vi "G#Object_NewObject.vi"(0 "reference in":refnum<class "G#Object.lvclass">, 1 "object name (\"\")":string, 2 "user counter (T)":bool=TRUE, 3 "no registration (F)":bool, 5 "error in (no error)":errorcluster, 6 "create method":T1) -> (14 "reference out":refnum<class "G#Object.lvclass">, 15 "created new?":bool, 19 "error out":errorcluster)   [LabVIEW 2020, in "G#Object.lvclass"]
doc: "Creates a new object and registers it."
uses:
  <vilib>/addons/_AddQ/G#Object/G#Object.lvclass
  <vilib>/addons/_AddQ/G#Object/utils/G#Object_CreateMethod.ctl
  <vilib>/addons/_AddQ/G#Object/utils/G#Object_State.ctl
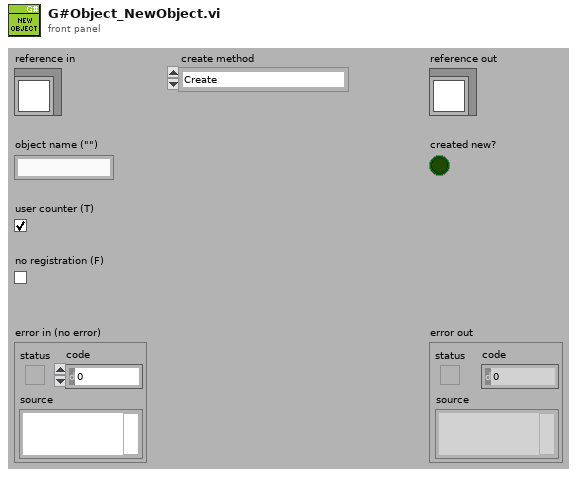
[diagram p1: front panel]
types:
  T1 = typedef "G#Object.lvclass/G#Object_CreateMethod.ctl" = enum16{"Create", "Create or look up existing", "Look up existing"}
  T2 = typedef "G#Object.lvclass/G#Object_State.ctl" = enum16{"Clear", "Create", "Delete", "Get class attributes", "Class hierarchy", "Get attribute value", "Set attribute value"}
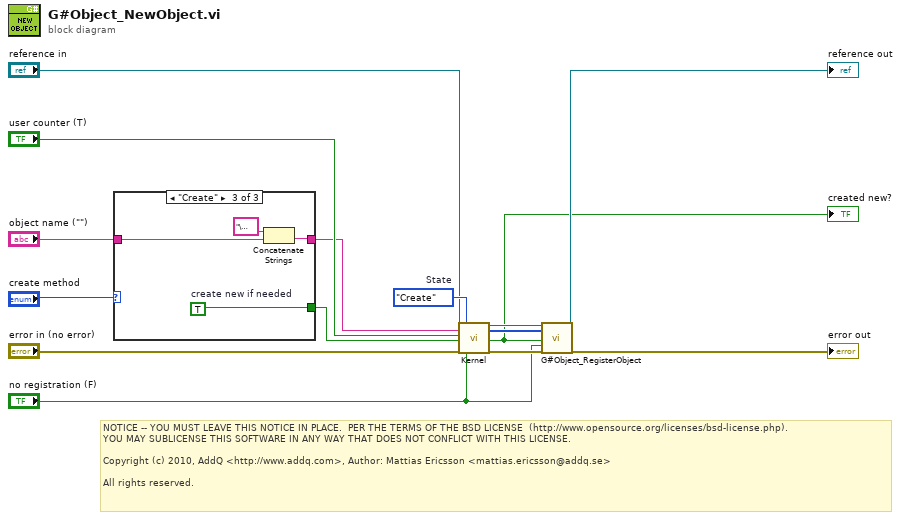
[diagram p0: block diagram]
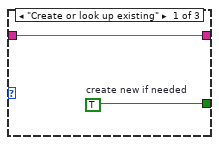
[diagram p2: hidden frame]
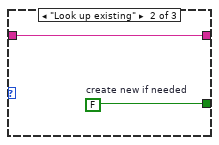
[diagram p3: hidden frame]
diagram:
  w13 = G#Object_State."Create"  # State
  # "NOTICE -- YOU MUST LEAVE THIS NOTICE IN PLACE.  PER THE TERMS OF THE BSD LICENSE  (http://www.opensource.org/licenses/bsd-license.php).\nYOU MAY SUBLICENSE THIS SOFTWARE IN ANY WAY THAT DOES NOT CONFLICT WITH THIS LICENSE.\n\nCopyright (c) 2010, AddQ <http://www.addq.com>, Author: Mattias Ericsson <mattias.ericsson@addq.se>\n\nAll rights reserved."
  n1 = case shown="\"Create\"" "create method" {
    tunnel: "object name (\"\")" -> [w17 w19 w21]
    tunnel: [w17 w19 w22] -> w9
    tunnel: [w16 w18 w23] -> w8
    frame "Create or look up existing" {
      w16 = TRUE  # create new if needed
    }
    frame "Look up existing" {
      w18 = FALSE  # create new if needed
    }
    frame "Create" {
      w23 = TRUE  # create new if needed
      n2 = Concatenate Strings("\u0000" ("string"), w21) -> (w22:string)
    }
  }
  n3 = call-dynamic "Kernel.vi"("reference in"="reference in", "object name"=w9, "option 1"="user counter (T)", "option 2"=w8, "error in (no error)"="error in (no error)", "state"=w13, "option 3"="no registration (F)") -> ("reference out"=w5:refnum<class "G#Object.lvclass">, "attribute refs"=w2:u32[], "output 1"=w1:bool, "error out"=w7:errorcluster)  [unwired: 4 in, 5 out]
  "created new?" <- w1
  n4 = call <vilib>:"G#Object_RegisterObject.vi"("reference in"=w5, "attribute refs"=w2, "created new"=w1, "no registration"="no registration (F)", "error in (no error)"=w7) -> ("reference out"=→"reference out":refnum<class "G#Object.lvclass">, "error out"=→"error out":errorcluster)  [unwired: 13 in]
